vi "Aurora Writer (Single Port).vi"(0 "input data":bool[](array[boolean]), 2 "AXI4-Stream Writer FXP64x4":T1, 9 "input valid":bool) -> (14 "ready for input":bool)   [LabVIEW 2019]
uses:
  AXI4-Stream Writer FXP64x4 Resources.ctl
  <vilib>/rvi/eio/common/nirviEmuTemplateMethod_errors.vi
  <vilib>/eio/EIONode/EIONode.xnode
  <instrlib>/_niInstr/Basic Elements/v1/FPGA/niInstr Basic Elements v1 FPGA.lvlib
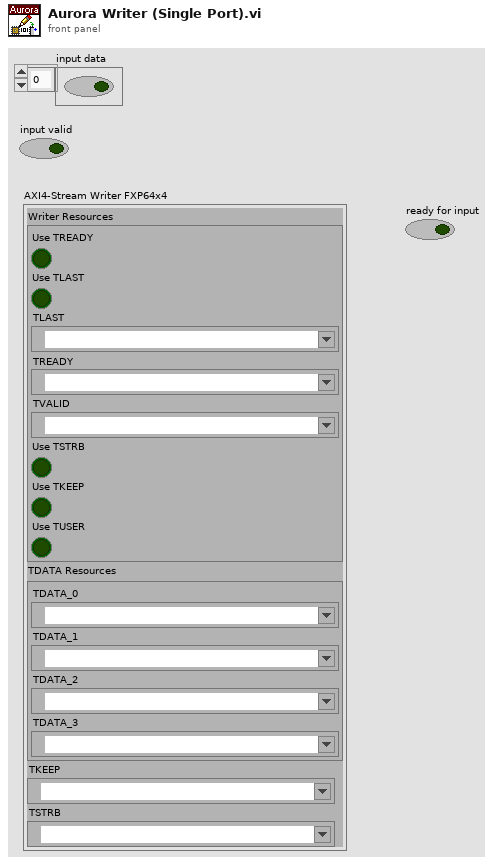
[diagram p1: front panel]
types:
  T1 = typedef "AXI4-Stream Writer FXP64x4 Resources.ctl" = cluster{"Writer Resources":cluster{"Use TREADY":bool, "Use TLAST":bool, "TLAST":refnum<k21>, "TREADY":refnum<k21>, "TVALID":refnum<k21>, "Use TSTRB":bool, "Use TKEEP":bool, "Use TUSER":bool}, "TDATA Resources":cluster{"TDATA_0":refnum<k21>, "TDATA_1":refnum<k21>, "TDATA_2":refnum<k21>, "TDATA_3":refnum<k21>}, "TKEEP":refnum<k21>, "TSTRB":refnum<k21>}
  T2 = cluster{"TDATA Width":i16, "TKEEP Width":i16, "TSTRB Width":i16, "TUSER Width":i16}
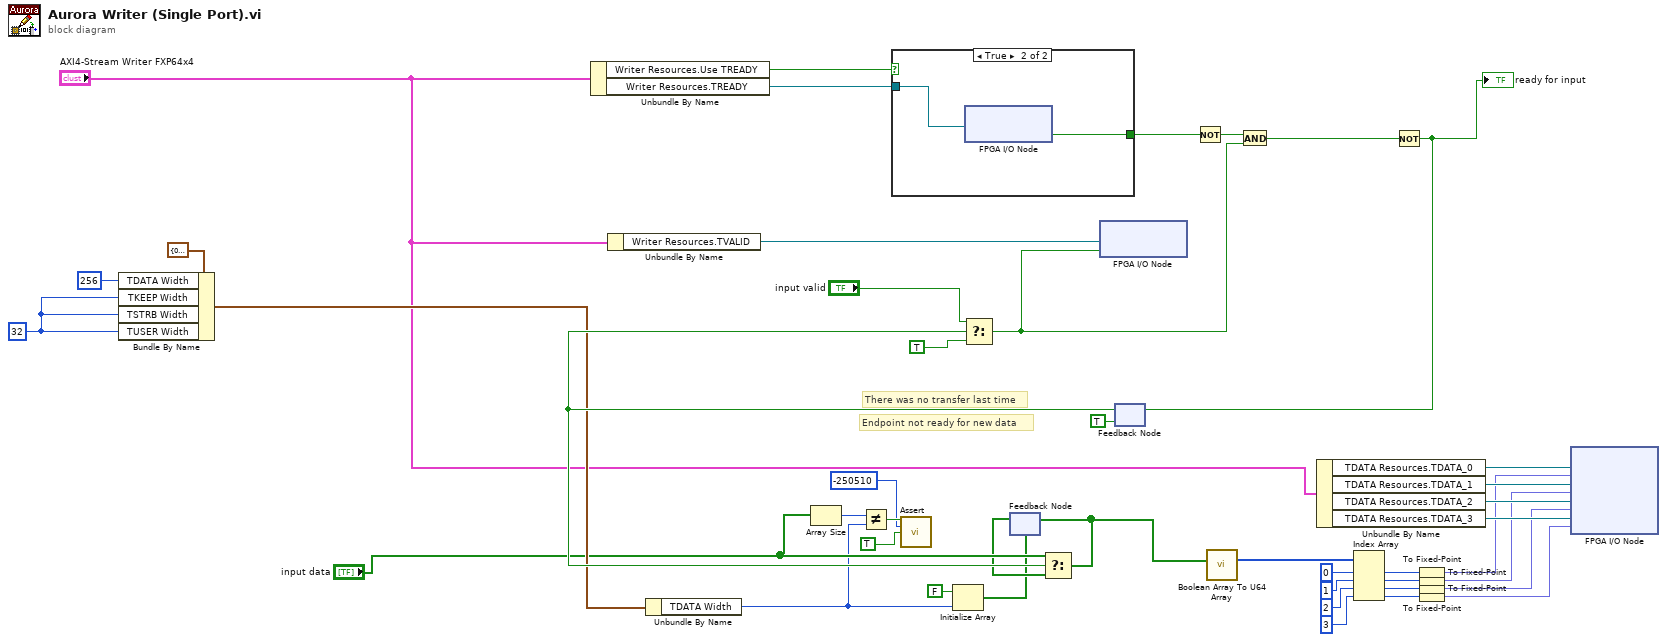
[diagram p0: block diagram]
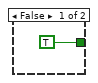
[diagram p2: hidden frame]
diagram:
  w34 = i16 32 ("TKEEP Width (Bits)")
  # "Endpoint not ready for new data"
  # "There was no transfer last time"
  n1 = Bundle By Name(cluster=T2 {"TDATA Width"=0, "TKEEP Width"=0, "TSTRB Width"=0, "TUSER Width"=0} ("port widths"), "TDATA Width"=i16 256 ("TDATA Width (Bits)"), "TKEEP Width"=w34, "TSTRB Width"=w34, "TUSER Width"=w34) -> (w31:T2)
  n2 = Unbundle By Name("AXI4-Stream Writer FXP64x4") -> ("Writer Resources.Use TREADY"=w44:bool, "Writer Resources.TREADY"=w42:refnum<k21>)
  n3 = Unbundle By Name("AXI4-Stream Writer FXP64x4") -> ("Writer Resources.TVALID"=w37:refnum<k21>)
  n4 = Unbundle By Name(w31) -> ("TDATA Width"=w20:i16)
  n5 = Array Size(array="input data") -> (size(s)=w24:i32)
  n6 = Not Equal?(x=w24, y=w20) -> (x != y?=w23:bool)
  n7 = case shown="True" w44 {
    tunnel: w42 -> [_ w47]
    tunnel: [TRUE ("I/O Item") w46] -> w39
    frame False {
    }
    frame True {
      n8 = xnode "FPGA I/O Node"("FPGA I/O In"=w47) -> ("I/O Item"=w46:bool)  [unwired: 1 out]
    }
  }
  n9 = call <instrlib>:"Assert.vi"("assert"=w23, "error code"=-250510, "enable show error"=TRUE) -> ()  [unwired: 13 in]
  n10 = Initialize Array(FALSE ("TLAST Value"), w20) -> (w25:bool[])
  n11 = feedback #1(w25) -> (w27:bool[])
  n12 = feedback #2(TRUE) -> (w35:bool)
  n13 = Select(t="input valid", s=w35, f=TRUE) -> (s? t:f=w36:bool)
  n14 = Select(t="input data", s=w35, f=w27) -> (s? t:f=w2:bool[])
  n15 = feedback-in #1(w2) -> ()
  n16 = xnode "FPGA I/O Node"("I/O Item"=w36, "FPGA I/O In"=w37) -> ()  [unwired: 1 out]
  n17 = Not(x=w39) -> (.not. x?=w40:bool)
  n18 = call "Boolean Array To U64 Array.vi"("data in"=w2) -> ("data out"=w1:u64[])  [unwired: 14 in]
  n19 = And(x=w40, y=w36) -> (x .and. y?=w41:bool)
  n20 = Unbundle By Name("AXI4-Stream Writer FXP64x4") -> ("TDATA Resources.TDATA_0"=w18:refnum<k21>, "TDATA Resources.TDATA_1"=w17:refnum<k21>, "TDATA Resources.TDATA_2"=w14:refnum<k21>, "TDATA Resources.TDATA_3"=w13:refnum<k21>)
  n21 = Index Array(array=w1, index #1=0 ("index"), index #2=1 ("index"), index #3=2 ("index"), index #4=3 ("index")) -> (element #1=w10:u64, element #2=w9:u64, element #3=w8:u64, element #4=w7:u64)
  n22 = Not(x=w41) -> (.not. x?=w29:bool)
  "ready for input" <- w29
  n23 = feedback-in #2(w29) -> ()
  n24 = To Fixed-Point(number=w10) -> (fixed-point=w6:fxp<+,64,64>)  [unwired: 1 in]
  n25 = To Fixed-Point(number=w9) -> (fixed-point=w5:fxp<+,64,64>)  [unwired: 1 in]
  n26 = To Fixed-Point(number=w8) -> (fixed-point=w4:fxp<+,64,64>)  [unwired: 1 in]
  n27 = To Fixed-Point(number=w7) -> (fixed-point=w3:fxp<+,64,64>)  [unwired: 1 in]
  n28 = xnode "FPGA I/O Node"("I/O Item"=w6, "FPGA I/O In"=w18, "I/O Item"=w5, "FPGA I/O In"=w17, "I/O Item"=w4, "FPGA I/O In"=w14, "I/O Item"=w3, "FPGA I/O In"=w13) -> ()  [unwired: 4 out]
